vi "Simulation-3 (Shift Register)_B220061.vi"() -> ()   [LabVIEW 2021]
panel:
  out "Array 2":i32[](array[numeric])
  out "Numeric 2":i32
  out "x + y":i32
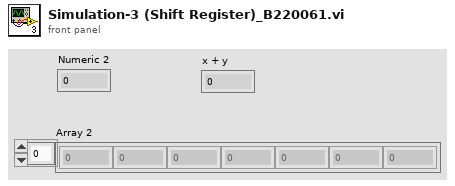
[diagram p1: front panel]
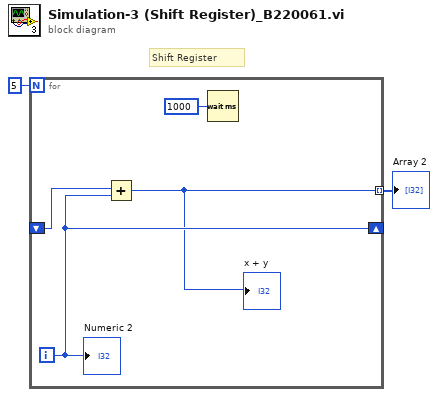
[diagram p0: block diagram]
diagram:
  # "Shift Register"
  n1 = for {
    N: 5 -> [_]
    shift-right: [w4] -> _
    shift-left: _ -> [w5]
    tunnel: [w3] -> w1 mode=indexing
    i -> [w4]
    n2 = Add(x=w5, y=w4) -> (x+y=w3:i32)
    "x + y" <- w3
    n3 = Wait (ms)(milliseconds to wait=u32 1000) -> ()  [unwired: 1 out]
    "Numeric 2" <- w4
  }
  "Array 2" <- w1
